vi "Untitled 2.vi"() -> ()   [LabVIEW 2018]
uses:
  <vilib>/Instr/_visa.llb/VISA Configure Serial Port (Instr).vi
panel:
  out "?":string
  in  "?":T1(tab)
  in  "IZQUIERDA":bool
  in  "ADELANTE":bool
  in  "DERECHA":bool
  in  "ATRAS":bool
  in  "automatico":bool
  in  "Slide":i32(slide) scale=0.0..255.0
  in  "on/off":bool
  out "led":bool
  out "Boolean":bool
  in  "?":bool
  in  "VISA resource name":refnum<visa-resource-name>
  # "FRENO"
  # "VELOCIDAD"
  # "OF"
  # "ON"
  # "OFF"
  # "DIRECCIÓN"
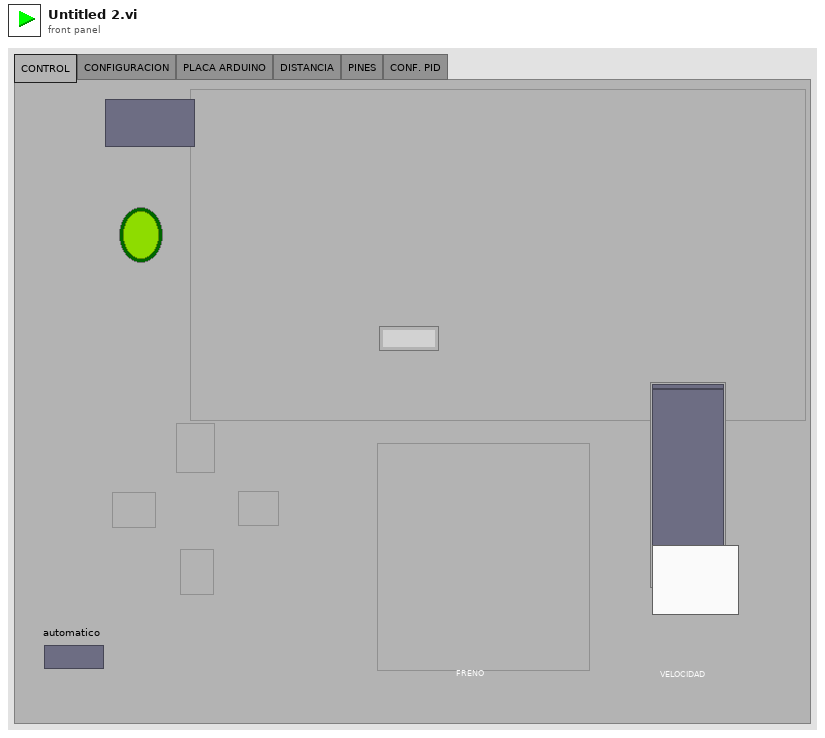
[diagram p1: front panel]
types:
  T1 = enum32{"CONTROL", "CONFIGURACION", "PLACA ARDUINO", "DISTANCIA", "PINES", "CONF. PID"}
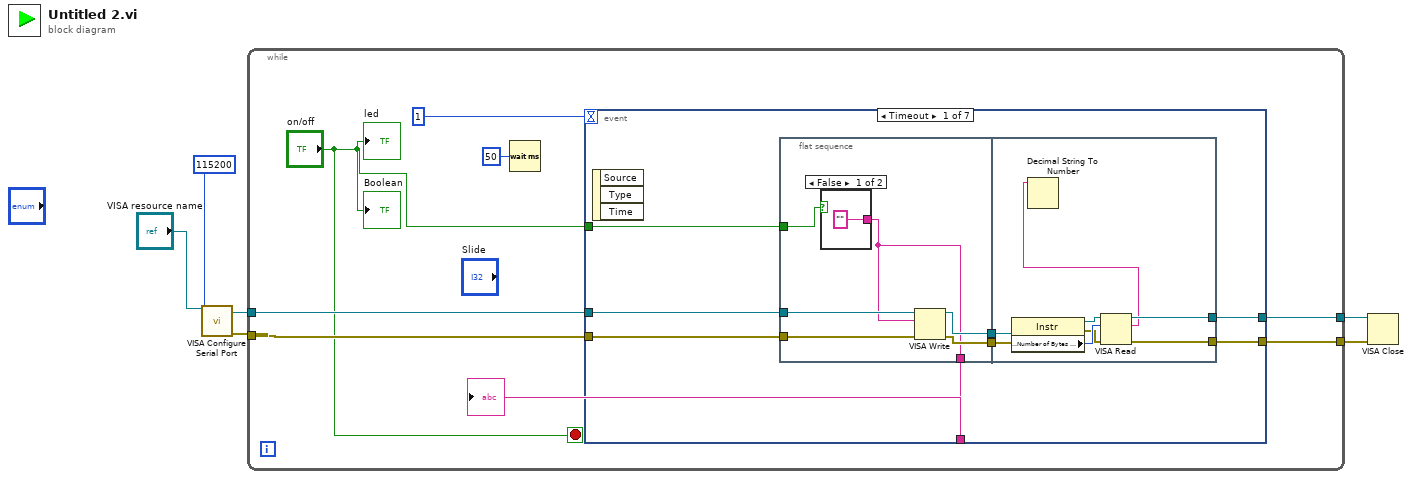
[diagram p0: block diagram]
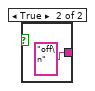
[diagram p2: hidden frame]
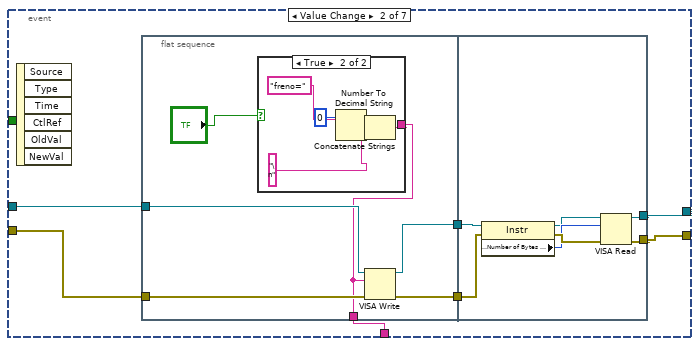
[diagram p3: hidden frame]
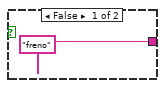
[diagram p4: hidden frame]
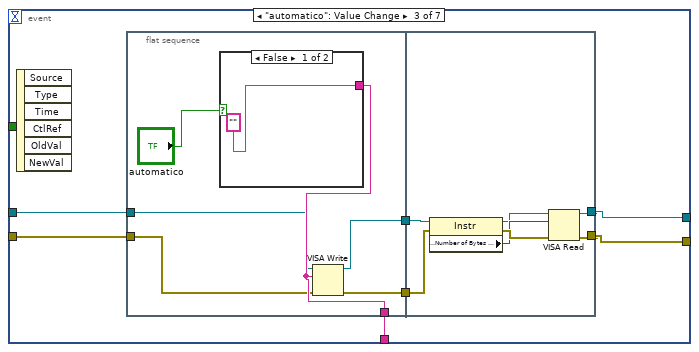
[diagram p5: hidden frame]
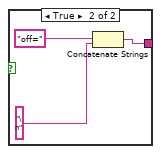
[diagram p6: hidden frame]
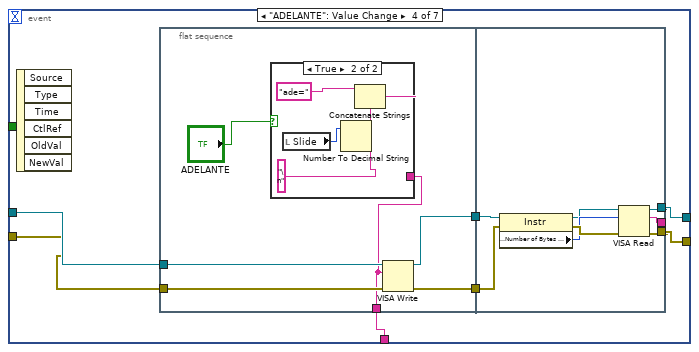
[diagram p7: hidden frame]
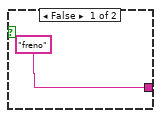
[diagram p8: hidden frame]
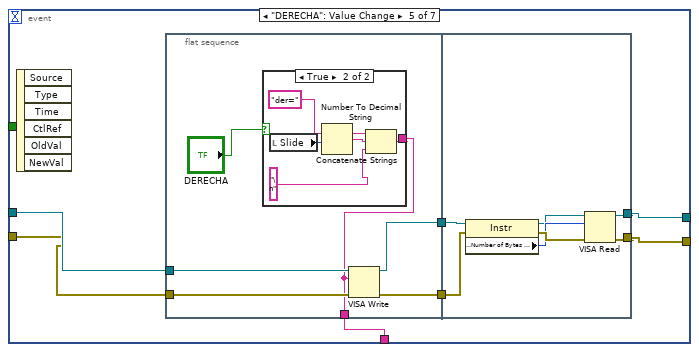
[diagram p9: hidden frame]
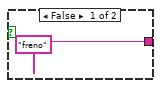
[diagram p10: hidden frame]
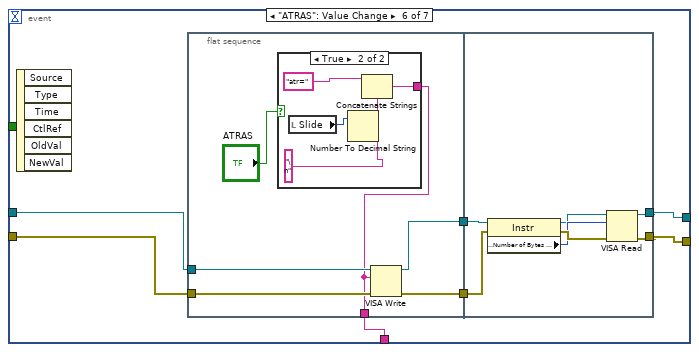
[diagram p11: hidden frame]
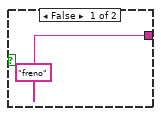
[diagram p12: hidden frame]
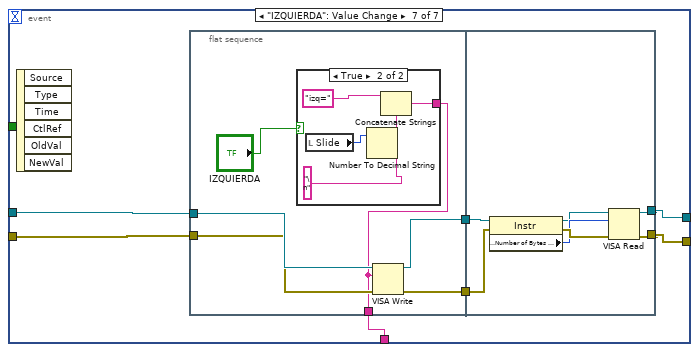
[diagram p13: hidden frame]
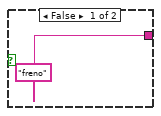
[diagram p14: hidden frame]
diagram:
  n1 = call-poly "VISA Configure Serial Port"("VISA resource name"="VISA resource name", "baud rate (9600)"=u32 115200) -> ("VISA resource name out"=w4:refnum<visa-resource-name>, "error out"=w3:errorcluster)  [unwired: 12 in]
  n2 = while {
    tunnel: w4 -> [w12]
    tunnel: w3 -> [w13]
    tunnel: [w10] -> w2
    tunnel: [w11] -> w1
    stop <- "on/off" stop-if-true
    n3 = Wait (ms)(milliseconds to wait=u32 50) -> ()  [unwired: 1 out]
    n4 = event shown="[0] Timeout" {
      selector: _ -> [_ _ _ _ _ _ _]
      dyn-events: _ -> [_ _ _ _ _ _ _]
      timeout: 1 -> [_ _ _ _ _ _ _]
      tunnel: w12 -> [w20 w43 w66 w93 w120 w144 w172]
      tunnel: w13 -> [w19 w42 w65 w92 w119 w143 w171]
      tunnel: [w18 w40 w68 w91 w118 w146 w170] -> w10
      tunnel: [w17 w41 w67 w90 w117 w145 w169] -> w11
      tunnel: [w16 w39 w69 w89 w116 w142 w168] -> w9
      tunnel: "on/off" -> [w15 _ _ _ _ _ _]
      event Timeout {
        n5 = event-data() -> ()  [unwired: 1 in, 3 out]
        n6 = flat-sequence {
          tunnel: [w28] -> w22
          tunnel: [w27] -> w21
          tunnel: w20 -> [w26]
          tunnel: w19 -> [w25]
          tunnel: [w24] -> w16
          tunnel: w15 -> [w23]
          tunnel: w22 -> [w35]
          tunnel: w21 -> [w34]
          tunnel: [w33] -> w17
          tunnel: [w32] -> w18
          frame #0 {
            n7 = case shown="False" w23 {
              tunnel: ["" "off\n"] -> w24
              frame False {
              }
              frame True {
              }
            }
            n8 = VISA Write(VISA resource name=w26, write buffer=w24, error in (no error)=w25) -> (VISA resource name out=w28:refnum<visa-resource-name>, error out=w27:errorcluster)  [unwired: 1 out]
          }
          frame #1 {
            n9 = property class="Instr"(reference=w35, error in=w34) -> (reference out=w36:refnum<visa-resource-name>, error out=w37:errorcluster, "Serial Settings:Number of Bytes at Serial Port"=w38:u32)
            n10 = VISA Read(VISA resource name=w36, byte count=w38, error in (no error)=w37) -> (VISA resource name out=w32:refnum<visa-resource-name>, read buffer=w31:string, error out=w33:errorcluster)  [unwired: 1 out]
            n11 = Decimal String To Number(string=w31) -> ()  [unwired: 2 in, 2 out]
          }
        }
      }
      event Value Change {
        n12 = event-data() -> ()  [unwired: 1 in, 6 out]
        n13 = flat-sequence {
          tunnel: [w51] -> w45
          tunnel: [w50] -> w44
          tunnel: w43 -> [w49]
          tunnel: w42 -> [w48]
          tunnel: [w46] -> w39
          tunnel: w45 -> [w61]
          tunnel: w44 -> [w60]
          tunnel: [w59] -> w40
          tunnel: [w58] -> w41
          frame #0 {
            n14 = case shown="True" "?" {
              tunnel: ["freno" w54] -> w46
              frame False {
              }
              frame True {
                n15 = Number To Decimal String(number=0) -> (decimal integer string=w57:string)  [unwired: 1 in]
                n16 = Concatenate Strings("freno=", w57, "\n") -> (w54:string)
              }
            }
            n17 = VISA Write(VISA resource name=w49, write buffer=w46, error in (no error)=w48) -> (VISA resource name out=w51:refnum<visa-resource-name>, error out=w50:errorcluster)  [unwired: 1 out]
          }
          frame #1 {
            n18 = property class="Instr"(reference=w61, error in=w60) -> (reference out=w62:refnum<visa-resource-name>, error out=w64:errorcluster, "Serial Settings:Number of Bytes at Serial Port"=w63:u32)
            n19 = VISA Read(VISA resource name=w62, byte count=w63, error in (no error)=w64) -> (VISA resource name out=w59:refnum<visa-resource-name>, error out=w58:errorcluster)  [unwired: 2 out]
          }
        }
      }
      event "automatico": Value Change {
        n20 = event-data() -> ()  [unwired: 1 in, 6 out]
        n21 = flat-sequence {
          tunnel: [w77] -> w71
          tunnel: [w76] -> w70
          tunnel: [w75] -> w69
          tunnel: w66 -> [w74]
          tunnel: w65 -> [w73]
          tunnel: w71 -> [w85]
          tunnel: w70 -> [w84]
          tunnel: [w83] -> w68
          tunnel: [w82] -> w67
          frame #0 {
            n22 = case shown="False" "automatico" {
              tunnel: ["" w81] -> w75
              frame False {
              }
              frame True {
                n23 = Concatenate Strings("off=", "\n") -> (w81:string)
              }
            }
            n24 = VISA Write(VISA resource name=w74, write buffer=w75, error in (no error)=w73) -> (VISA resource name out=w77:refnum<visa-resource-name>, error out=w76:errorcluster)  [unwired: 1 out]
          }
          frame #1 {
            n25 = property class="Instr"(reference=w85, error in=w84) -> (reference out=w86:refnum<visa-resource-name>, error out=w88:errorcluster, "Serial Settings:Number of Bytes at Serial Port"=w87:u32)
            n26 = VISA Read(VISA resource name=w86, byte count=w87, error in (no error)=w88) -> (VISA resource name out=w83:refnum<visa-resource-name>, error out=w82:errorcluster)  [unwired: 2 out]
          }
        }
      }
      event "ADELANTE": Value Change {
        n27 = event-data() -> ()  [unwired: 1 in, 6 out]
        n28 = flat-sequence {
          tunnel: [w101] -> w95
          tunnel: [w100] -> w94
          tunnel: w93 -> [w99]
          tunnel: w92 -> [w98]
          tunnel: [w96] -> w89
          tunnel: w95 -> [w112]
          tunnel: w94 -> [w111]
          tunnel: [w110] -> w91
          tunnel: [w109] -> w90
          tunnel: [w108] -> _
          frame #0 {
            n29 = case shown="True" "ADELANTE" {
              tunnel: ["freno" w104] -> w96
              frame False {
              }
              frame True {
                n30 = local read "Slide"() -> (w103:i32)
                n31 = Number To Decimal String(number=w103) -> (decimal integer string=w107:string)  [unwired: 1 in]
                n32 = Concatenate Strings("ade=", w107, "\n") -> (w104:string)
              }
            }
            n33 = VISA Write(VISA resource name=w99, write buffer=w96, error in (no error)=w98) -> (VISA resource name out=w101:refnum<visa-resource-name>, error out=w100:errorcluster)  [unwired: 1 out]
          }
          frame #1 {
            n34 = property class="Instr"(reference=w112, error in=w111) -> (reference out=w113:refnum<visa-resource-name>, error out=w115:errorcluster, "Serial Settings:Number of Bytes at Serial Port"=w114:u32)
            n35 = VISA Read(VISA resource name=w113, byte count=w114, error in (no error)=w115) -> (VISA resource name out=w110:refnum<visa-resource-name>, read buffer=w108:string, error out=w109:errorcluster)  [unwired: 1 out]
          }
        }
      }
      event "DERECHA": Value Change {
        n36 = event-data() -> ()  [unwired: 1 in, 6 out]
        n37 = flat-sequence {
          tunnel: [w128] -> w122
          tunnel: [w127] -> w121
          tunnel: w120 -> [w126]
          tunnel: w119 -> [w125]
          tunnel: [w123] -> w116
          tunnel: w122 -> [w138]
          tunnel: w121 -> [w137]
          tunnel: [w136] -> w118
          tunnel: [w135] -> w117
          frame #0 {
            n38 = case shown="True" "DERECHA" {
              tunnel: ["freno" w131] -> w123
              frame False {
              }
              frame True {
                n39 = local read "Slide"() -> (w130:i32)
                n40 = Number To Decimal String(number=w130) -> (decimal integer string=w134:string)  [unwired: 1 in]
                n41 = Concatenate Strings("der=", w134, "\n") -> (w131:string)
              }
            }
            n42 = VISA Write(VISA resource name=w126, write buffer=w123, error in (no error)=w125) -> (VISA resource name out=w128:refnum<visa-resource-name>, error out=w127:errorcluster)  [unwired: 1 out]
          }
          frame #1 {
            n43 = property class="Instr"(reference=w138, error in=w137) -> (reference out=w139:refnum<visa-resource-name>, error out=w141:errorcluster, "Serial Settings:Number of Bytes at Serial Port"=w140:u32)
            n44 = VISA Read(VISA resource name=w139, byte count=w140, error in (no error)=w141) -> (VISA resource name out=w136:refnum<visa-resource-name>, error out=w135:errorcluster)  [unwired: 2 out]
          }
        }
      }
      event "ATRAS": Value Change {
        n45 = event-data() -> ()  [unwired: 1 in, 6 out]
        n46 = flat-sequence {
          tunnel: [w154] -> w148
          tunnel: [w153] -> w147
          tunnel: w144 -> [w152]
          tunnel: w143 -> [w151]
          tunnel: [w149] -> w142
          tunnel: w148 -> [w164]
          tunnel: w147 -> [w163]
          tunnel: [w162] -> w146
          tunnel: [w161] -> w145
          frame #0 {
            n47 = case shown="True" "ATRAS" {
              tunnel: ["freno" w156] -> w149
              frame False {
              }
              frame True {
                n48 = local read "Slide"() -> (w157:i32)
                n49 = Number To Decimal String(number=w157) -> (decimal integer string=w160:string)  [unwired: 1 in]
                n50 = Concatenate Strings("atr=", w160, "\n") -> (w156:string)
              }
            }
            n51 = VISA Write(VISA resource name=w152, write buffer=w149, error in (no error)=w151) -> (VISA resource name out=w154:refnum<visa-resource-name>, error out=w153:errorcluster)  [unwired: 1 out]
          }
          frame #1 {
            n52 = property class="Instr"(reference=w164, error in=w163) -> (reference out=w165:refnum<visa-resource-name>, error out=w167:errorcluster, "Serial Settings:Number of Bytes at Serial Port"=w166:u32)
            n53 = VISA Read(VISA resource name=w165, byte count=w166, error in (no error)=w167) -> (VISA resource name out=w162:refnum<visa-resource-name>, error out=w161:errorcluster)  [unwired: 2 out]
          }
        }
      }
      event "IZQUIERDA": Value Change {
        n54 = event-data() -> ()  [unwired: 1 in, 6 out]
        n55 = flat-sequence {
          tunnel: [w180] -> w174
          tunnel: [w179] -> w173
          tunnel: w172 -> [w178]
          tunnel: w171 -> [w177]
          tunnel: [w175] -> w168
          tunnel: w174 -> [w190]
          tunnel: w173 -> [w189]
          tunnel: [w188] -> w170
          tunnel: [w187] -> w169
          frame #0 {
            n56 = case shown="True" "IZQUIERDA" {
              tunnel: ["freno" w183] -> w175
              frame False {
              }
              frame True {
                n57 = local read "Slide"() -> (w182:i32)
                n58 = Number To Decimal String(number=w182) -> (decimal integer string=w186:string)  [unwired: 1 in]
                n59 = Concatenate Strings("izq=", w186, "\n") -> (w183:string)
              }
            }
            n60 = VISA Write(VISA resource name=w178, write buffer=w175, error in (no error)=w177) -> (VISA resource name out=w180:refnum<visa-resource-name>, error out=w179:errorcluster)  [unwired: 1 out]
          }
          frame #1 {
            n61 = property class="Instr"(reference=w190, error in=w189) -> (reference out=w191:refnum<visa-resource-name>, error out=w193:errorcluster, "Serial Settings:Number of Bytes at Serial Port"=w192:u32)
            n62 = VISA Read(VISA resource name=w191, byte count=w192, error in (no error)=w193) -> (VISA resource name out=w188:refnum<visa-resource-name>, error out=w187:errorcluster)  [unwired: 2 out]
          }
        }
      }
    }
    "?" <- w9
    "led" <- "on/off"
    "Boolean" <- "on/off"
  }
  n63 = VISA Close(VISA resource name=w2, error in (no error)=w1) -> ()  [unwired: 1 out]
